vi "Revisión_VFD.vi"(5 "Fabricante":u32, 6 "Modbus":T1, 7 "Iteración (In)":u32, 8 "Motor":T2, 9 "I/O":T3, 10 "Referencias":T4, 11 "Instancia Modbus":refnum<class "Modbus Master.lvclass">) -> (0 "Error Modbus":errorcluster, 2 "Iteración (Out)":u32, 3 "Coincidentes":bool[](array[boolean]))   [LabVIEW 2013]
uses:
  <vilib>/NI/Modbus Library/API/Master/Modbus Master.lvclass
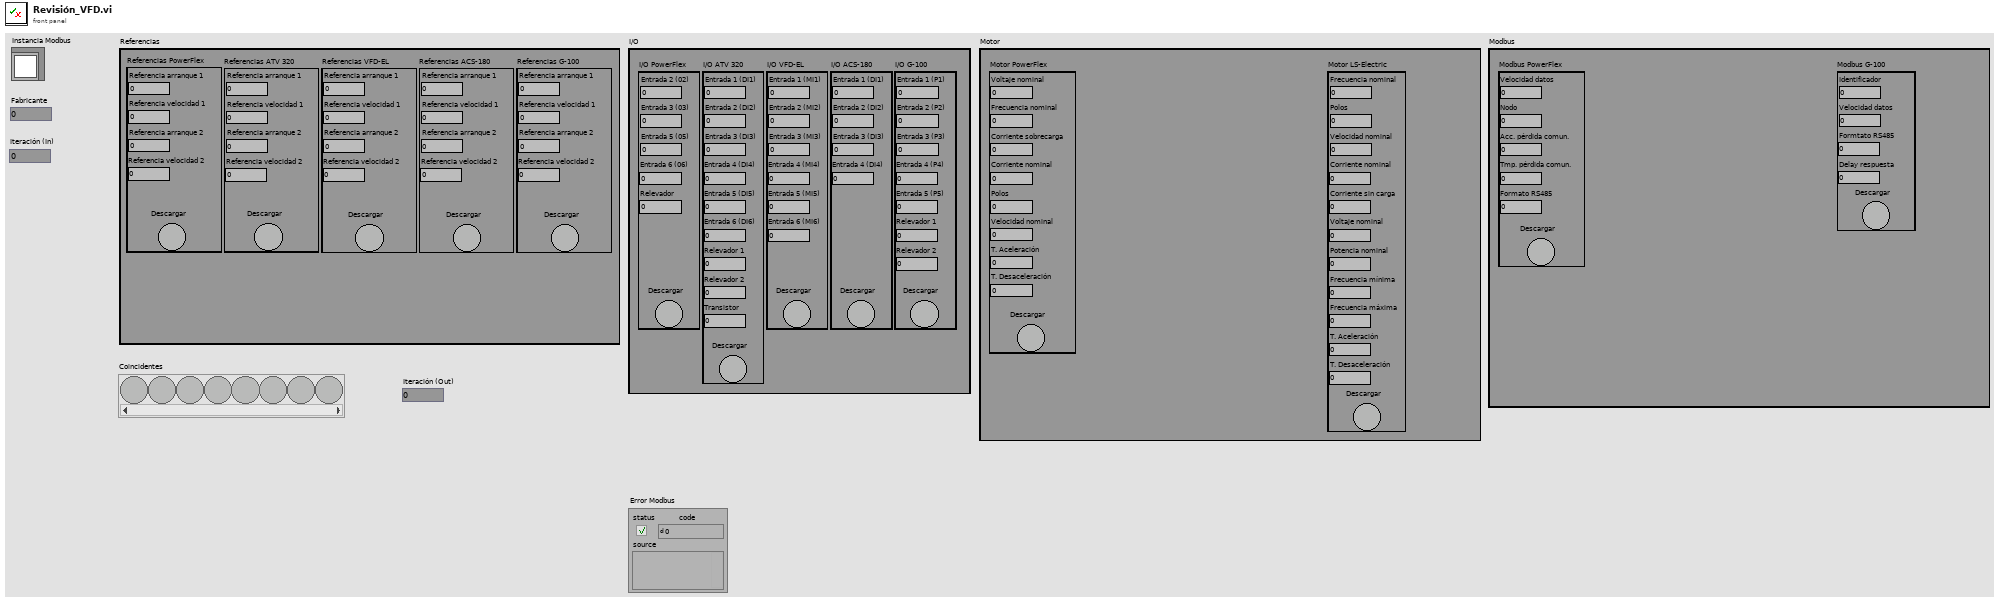
[diagram p1: front panel]
types:
  T1 = cluster{"Modbus PowerFlex":cluster{"Velocidad datos":u16, "Nodo":u16, "Acc. pérdida comun.":u16, "Tmp. pérdida comun.":u16, "Formato RS485":u16, "Descargar":bool}, "Modbus G-100":cluster{"Identificador":u16, "Velocidad datos":u16, "Formtato RS485":u16, "Delay respuesta":u16, "Descargar":bool}}
  T2 = cluster{"Motor PowerFlex":cluster{"Voltaje nominal":u16, "Frecuencia nominal":u16, "Corriente sobrecarga":dbl, "Corriente nominal":dbl, "Polos":u16, "Velocidad nominal":u16, "T. Aceleración":dbl, "T. Desaceleración":dbl, "Descargar":bool}, "Motor LS-Electric":cluster{"Frecuencia nominal":u16, "Polos":u16, "Velocidad nominal":u16, "Corriente nominal":dbl, "Corriente sin carga":dbl, "Voltaje nominal":u16, "Potencia nominal":u16, "Frecuencia mínima":dbl, "Frecuencia máxima":dbl, "T. Aceleración":dbl, "T. Desaceleración":dbl, "Descargar":bool}}
  T3 = cluster{"I/O PowerFlex":cluster{"Entrada 2 (02)":u16, "Entrada 3 (03)":u16, "Entrada 5 (05)":u16, "Entrada 6 (06)":u16, "Relevador":u16, "Descargar":bool}, "I/O ATV 320":cluster{"Entrada 1 (DI1)":u16, "Entrada 2 (DI2)":u16, "Entrada 3 (DI3)":u16, "Entrada 4 (DI4)":u16, "Entrada 5 (DI5)":u16, "Entrada 6 (DI6)":u16, "Relevador 1":u16, "Relevador 2":u16, "Transistor":u16, "Descargar":bool}, "I/O VFD-EL":cluster{"Entrada 1 (MI1)":u16, "Entrada 2 (MI2)":u16, "Entrada 3 (MI3)":u16, "Entrada 4 (MI4)":u16, "Entrada 5 (MI5)":u16, "Entrada 6 (MI6)":u16, "Descargar":bool}, "I/O ACS-180":cluster{"Entrada 1 (DI1)":u16, "Entrada 2 (DI2)":u16, "Entrada 3 (DI3)":u16, "Entrada 4 (DI4)":u16, "Descargar":bool}, "I/O G-100":cluster{"Entrada 1 (P1)":u16, "Entrada 2 (P2)":u16, "Entrada 3 (P3)":u16, "Entrada 4 (P4)":u16, "Entrada 5 (P5)":u16, "Relevador 1":u16, "Relevador 2":u16, "Descargar":bool}}
  T4 = cluster{"Referencias PowerFlex":cluster{"Referencia arranque 1":u16, "Referencia velocidad 1":u16, "Referencia arranque 2":u16, "Referencia velocidad 2":u16, "Descargar":bool}, "Referencias ATV 320":cluster{"Referencia arranque 1":u16, "Referencia velocidad 1":u16, "Referencia arranque 2":u16, "Referencia velocidad 2":u16, "Descargar":bool}, "Referencias VFD-EL":cluster{"Referencia arranque 1":u16, "Referencia velocidad 1":u16, "Referencia arranque 2":u16, "Referencia velocidad 2":u16, "Descargar":bool}, "Referencias ACS-180":cluster{"Referencia arranque 1":u16, "Referencia velocidad 1":u16, "Referencia arranque 2":u16, "Referencia velocidad 2":u16, "Descargar":bool}, "Referencias G-100":cluster{"Referencia arranque 1":u16, "Referencia velocidad 1":u16, "Referencia arranque 2":u16, "Referencia velocidad 2":u16, "Descargar":bool}}
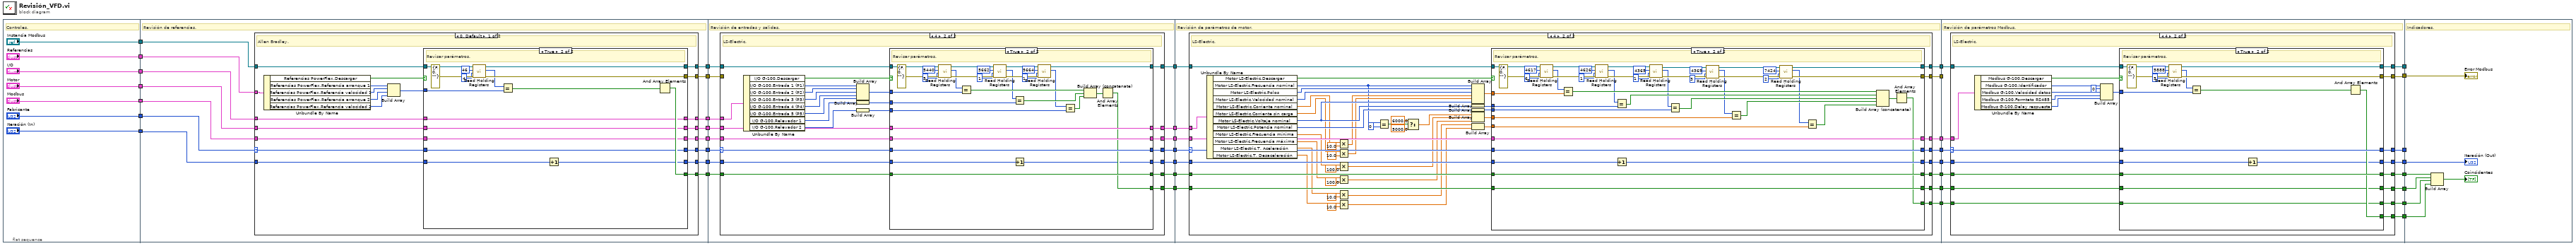
[diagram p0: block diagram]
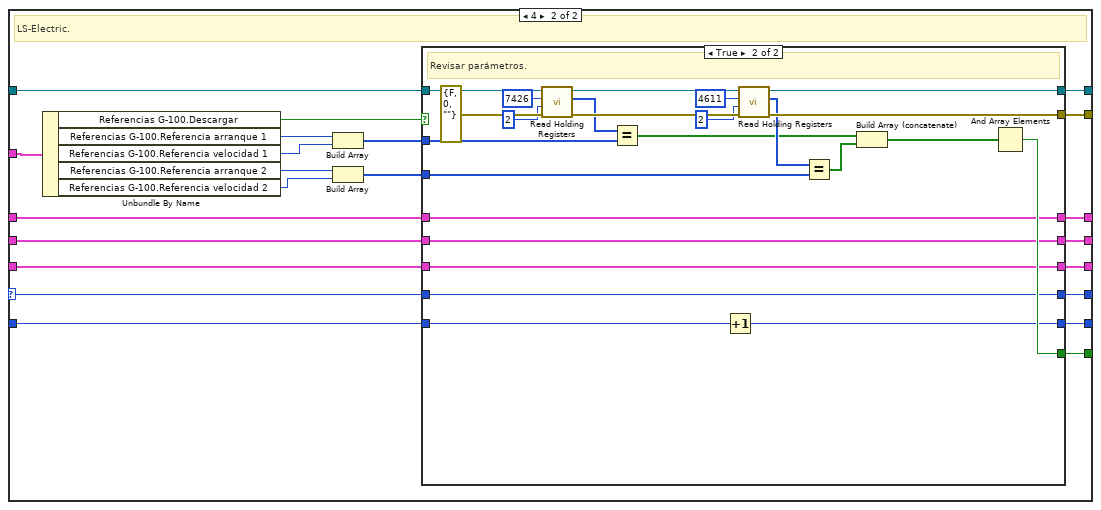
[diagram p3: hidden frame]
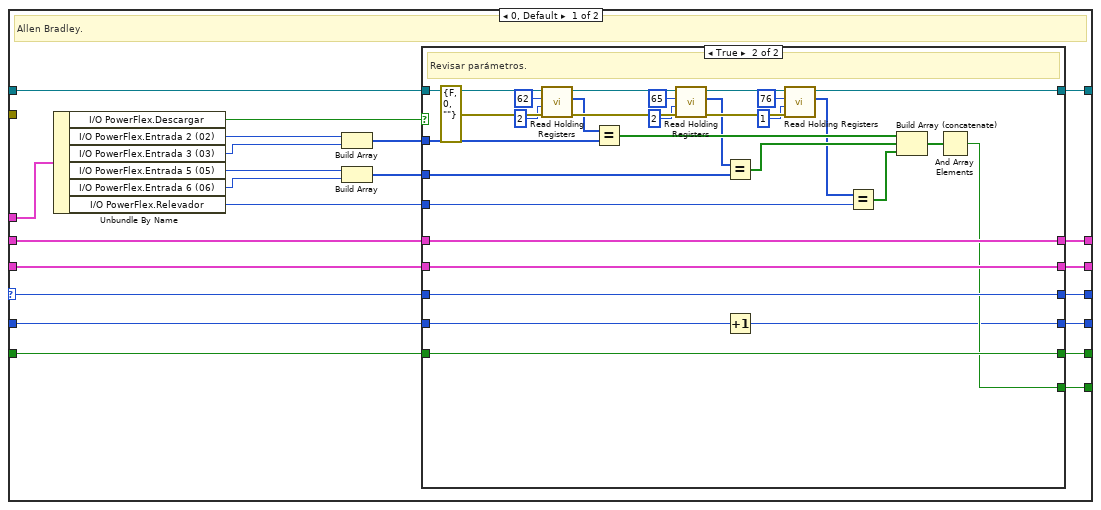
[diagram p5: hidden frame]
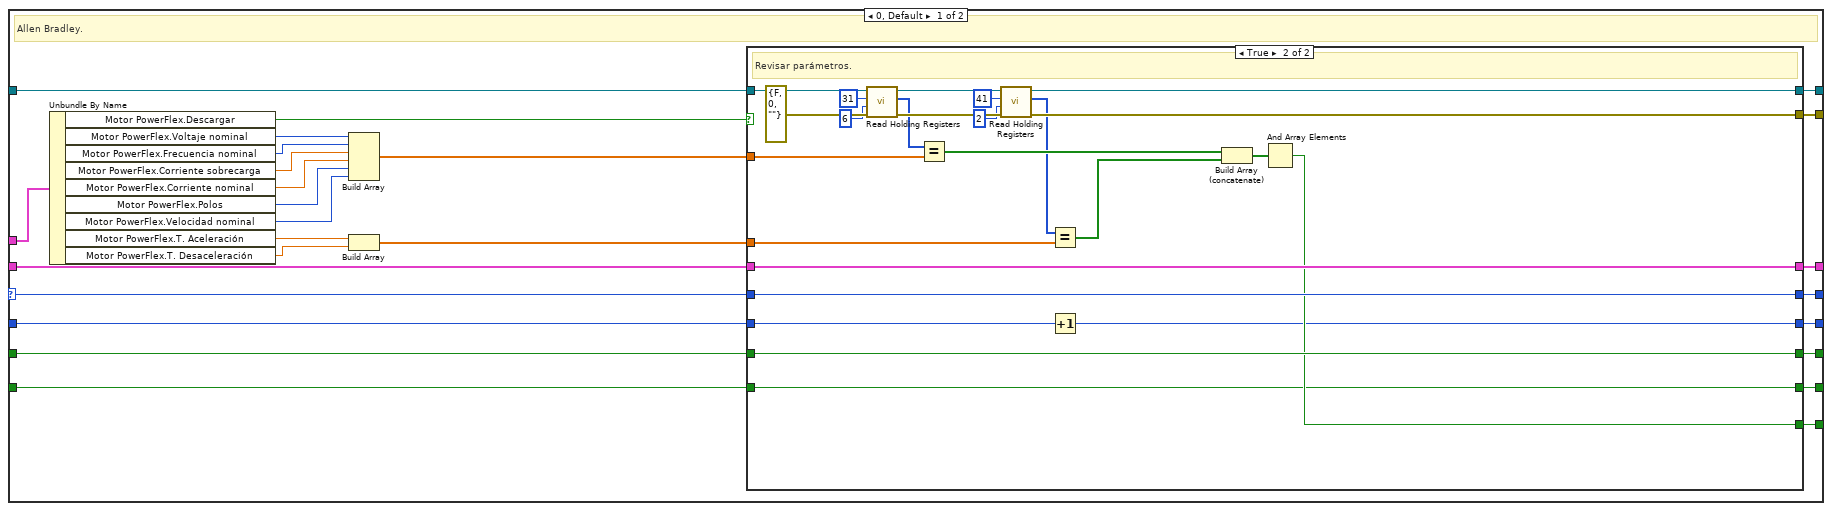
[diagram p8: hidden frame]
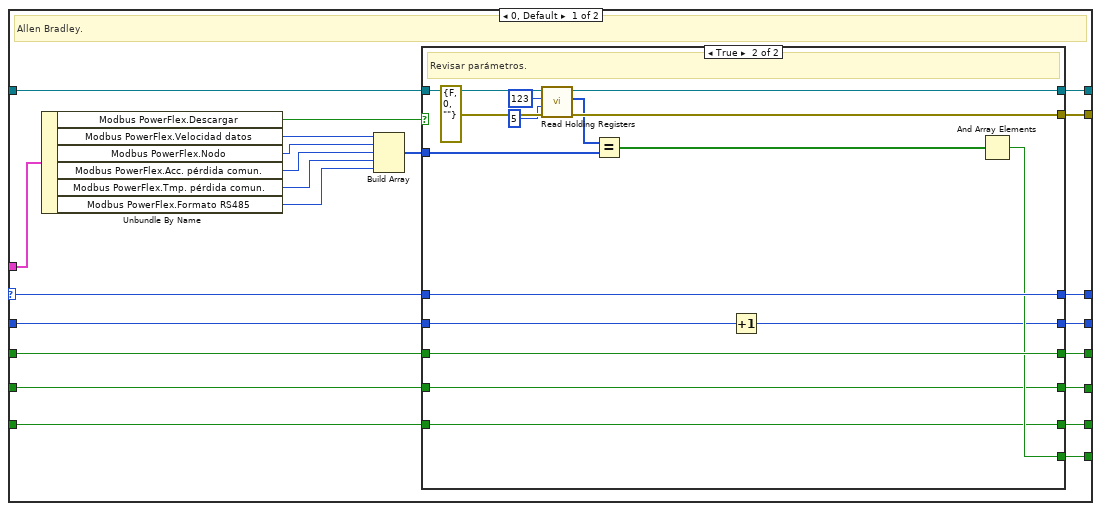
[diagram p11: hidden frame]
diagram:
  n1 = flat-sequence {
    tunnel: ["Instancia Modbus"] -> w38
    tunnel: ["Fabricante"] -> w37
    tunnel: ["Referencias"] -> w36
    tunnel: ["I/O"] -> w35
    tunnel: ["Motor"] -> w34
    tunnel: ["Modbus"] -> w33
    tunnel: ["Iteración (In)"] -> w6
    tunnel: w38 -> [w59]
    tunnel: w37 -> [w60]
    tunnel: w36 -> [w58]
    tunnel: w35 -> [w56]
    tunnel: w34 -> [w55]
    tunnel: w33 -> [w54]
    tunnel: [w57] -> w32
    tunnel: [w53] -> w31
    tunnel: [w52] -> w30
    tunnel: [w51] -> w29
    tunnel: [w50] -> w28
    tunnel: [w49] -> w27
    tunnel: [w48] -> w26
    tunnel: w6 -> [w47]
    tunnel: [w46] -> w5
    tunnel: w32 -> [w164]
    tunnel: w31 -> [w168]
    tunnel: w30 -> [w167]
    tunnel: w29 -> [w166]
    tunnel: w28 -> [w165]
    tunnel: w27 -> [w170]
    tunnel: w26 -> [w169]
    tunnel: [w163] -> w25
    tunnel: [w162] -> w24
    tunnel: [w161] -> w23
    tunnel: [w160] -> w22
    tunnel: [w159] -> w21
    tunnel: [w158] -> w20
    tunnel: w5 -> [w157]
    tunnel: [w156] -> w4
    tunnel: w25 -> [w303]
    tunnel: w24 -> [w302]
    tunnel: w23 -> [w301]
    tunnel: w22 -> [w300]
    tunnel: w21 -> [w299]
    tunnel: w20 -> [w304]
    tunnel: [w298] -> w19
    tunnel: [w297] -> w18
    tunnel: [w296] -> w17
    tunnel: [w295] -> w16
    tunnel: [w294] -> w15
    tunnel: [w293] -> w14
    tunnel: [w292] -> w13
    tunnel: w4 -> [w291]
    tunnel: [w290] -> w3
    tunnel: w19 -> [_]
    tunnel: w18 -> [w475]
    tunnel: w17 -> [w474]
    tunnel: w16 -> [w473]
    tunnel: w15 -> [w472]
    tunnel: w14 -> [w471]
    tunnel: w13 -> [w470]
    tunnel: [w469] -> w12
    tunnel: [w468] -> w11
    tunnel: [w467] -> w10
    tunnel: [w466] -> w9
    tunnel: [w465] -> w8
    tunnel: [w464] -> w7
    tunnel: w3 -> [w463]
    tunnel: [w462] -> w2
    tunnel: [w461] -> w1
    tunnel: w12 -> [_]
    tunnel: w11 -> [w570]
    tunnel: w10 -> [w569]
    tunnel: w9 -> [w568]
    tunnel: w8 -> [w567]
    tunnel: w7 -> [w566]
    tunnel: w2 -> [w564]
    tunnel: w1 -> [_]
    frame #0 {
      # "Controles."
    }
    frame #1 {
      # "Revisión de referencias."
      n2 = case shown="0, Default" w60 {
        selector: w60 -> [w74 w118]
        tunnel: w59 -> [w81 w125]
        tunnel: w58 -> [w80 w124]
        tunnel: [w78 w122] -> w57
        tunnel: w56 -> [w77 w121]
        tunnel: w55 -> [w76 w120]
        tunnel: w54 -> [w75 w119]
        tunnel: [w73 w117] -> w53
        tunnel: [w72 w116] -> w52
        tunnel: [w71 w115] -> w51
        tunnel: [w70 w114] -> w50
        tunnel: [w69 w113] -> w49
        tunnel: [w68 w112] -> w48
        tunnel: w47 -> [w62 w108]
        tunnel: [w61 w107] -> w46
        frame 0, Default {
          # "Allen Bradley."
          n3 = Unbundle By Name(w80) -> ("Referencias PowerFlex.Descargar"=w79:bool, "Referencias PowerFlex.Referencia arranque 1"=w67:u16, "Referencias PowerFlex.Referencia velocidad 1"=w66:u16, "Referencias PowerFlex.Referencia arranque 2"=w65:u16, "Referencias PowerFlex.Referencia velocidad 2"=w64:u16)
          n4 = Build Array(w67, w66, w65, w64) -> (w63:u16[])
          n5 = case shown="True" w79 {
            tunnel: w81 -> [w87 w102]
            tunnel: [_ w96] -> w78
            tunnel: w77 -> [w84 w95]
            tunnel: w76 -> [w83 w94]
            tunnel: w75 -> [w82 w93]
            tunnel: w74 -> [w85 w92]
            tunnel: [w84 w95] -> w73
            tunnel: [w83 w94] -> w72
            tunnel: [w82 w93] -> w71
            tunnel: [w85 w92] -> w70
            tunnel: [w87 w91] -> w69
            tunnel: [_ w103] -> w68
            tunnel: w63 -> [_ w90]
            tunnel: w62 -> [w86 w89]
            tunnel: [w86 w88] -> w61
            frame False {
              # "Nada."
            }
            frame True {
              # "Revisar parámetros."
              n6 = call-dynamic "Read Holding Registers.vi"("error in"=errorcluster {"status"=FALSE, "code"=0, "source"=""}, "number of inputs"=u16 4, "starting address"=u16 46, "Modbus master in"=w102) -> ("error out"=w103:errorcluster, "register values"=w98:u16[], "Modbus master out"=w91:refnum<class "Modbus Master.lvclass">)  [unwired: 5 in]
              n7 = Equal?(x=w98, y=w90) -> (x = y?=w97:bool[])
              n8 = Increment(x=w89) -> (x+1=w88:u32)
              n9 = And Array Elements(Boolean array=w97) -> (logical AND=w96:bool)
            }
          }
        }
        frame 4 {
          # "LS-Electric."
          n10 = Unbundle By Name(w124) -> ("Referencias G-100.Descargar"=w123:bool, "Referencias G-100.Referencia arranque 1"=w111:u16, "Referencias G-100.Referencia velocidad 1"=w110:u16, "Referencias G-100.Referencia arranque 2"=w106:u16, "Referencias G-100.Referencia velocidad 2"=w105:u16)
          n11 = Build Array(w111, w110) -> (w109:u16[])
          n12 = Build Array(w106, w105) -> (w104:u16[])
          n13 = case shown="True" w123 {
            tunnel: w125 -> [w131 w154]
            tunnel: [_ w149] -> w122
            tunnel: w121 -> [w128 w148]
            tunnel: w120 -> [w127 w147]
            tunnel: w119 -> [w126 w146]
            tunnel: w118 -> [w129 w145]
            tunnel: [w128 w148] -> w117
            tunnel: [w127 w147] -> w116
            tunnel: [w126 w146] -> w115
            tunnel: [w129 w145] -> w114
            tunnel: [w131 w139] -> w113
            tunnel: [_ w138] -> w112
            tunnel: w109 -> [_ w144]
            tunnel: w108 -> [w130 w143]
            tunnel: [w130 w142] -> w107
            tunnel: w104 -> [_ w141]
            frame False {
              # "Nada."
            }
            frame True {
              # "Revisar parámetros."
              n14 = call-dynamic "Read Holding Registers.vi"("error in"=errorcluster {"status"=FALSE, "code"=0, "source"=""}, "number of inputs"=u16 2, "starting address"=u16 7426, "Modbus master in"=w154) -> ("error out"=w155:errorcluster, "register values"=w150:u16[], "Modbus master out"=w140:refnum<class "Modbus Master.lvclass">)  [unwired: 5 in]
              n15 = Equal?(x=w150, y=w144) -> (x = y?=w134:bool[])
              n16 = Increment(x=w143) -> (x+1=w142:u32)
              n17 = call-dynamic "Read Holding Registers.vi"("error in"=w155, "number of inputs"=u16 2, "starting address"=u16 4611, "Modbus master in"=w140) -> ("error out"=w138:errorcluster, "register values"=w135:u16[], "Modbus master out"=w139:refnum<class "Modbus Master.lvclass">)  [unwired: 5 in]
              n18 = Equal?(x=w135, y=w141) -> (x = y?=w133:bool[])
              n19 = Build Array (concatenate)(w134, w133) -> (w132:bool[])
              n20 = And Array Elements(Boolean array=w132) -> (logical AND=w149:bool)
            }
          }
        }
      }
    }
    frame #2 {
      # "Revisión de entradas y salidas."
      n21 = case shown="4" w165 {
        selector: w165 -> [w188 w249]
        tunnel: w170 -> [w192 w253]
        tunnel: w168 -> [w184 w245]
        tunnel: w167 -> [w190 w251]
        tunnel: w166 -> [w189 w250]
        tunnel: [w187 w248] -> w163
        tunnel: [w186 w247] -> w162
        tunnel: [w185 w246] -> w161
        tunnel: w169 -> [_ _]
        tunnel: w164 -> [w183 w244]
        tunnel: [w182 w243] -> w160
        tunnel: [w178 w239] -> w158
        tunnel: [w173 w237] -> w159
        tunnel: w157 -> [w172 w236]
        tunnel: [w171 w235] -> w156
        frame 0, Default {
          # "Allen Bradley."
          n22 = Unbundle By Name(w184) -> ("I/O PowerFlex.Descargar"=w191:bool, "I/O PowerFlex.Entrada 2 (02)"=w181:u16, "I/O PowerFlex.Entrada 3 (03)"=w180:u16, "I/O PowerFlex.Entrada 5 (05)"=w177:u16, "I/O PowerFlex.Entrada 6 (06)"=w176:u16, "I/O PowerFlex.Relevador"=w175:u16)
          n23 = Build Array(w181, w180) -> (w179:u16[])
          n24 = Build Array(w177, w176) -> (w174:u16[])
          n25 = case shown="True" w191 {
            tunnel: w192 -> [w198 w225]
            tunnel: w190 -> [w197 w221]
            tunnel: w189 -> [w196 w220]
            tunnel: w188 -> [w195 w219]
            tunnel: [w197 w221] -> w187
            tunnel: [w196 w220] -> w186
            tunnel: [w195 w219] -> w185
            tunnel: [w194 w218] -> w182
            tunnel: w183 -> [w194 w218]
            tunnel: w179 -> [_ w209]
            tunnel: [w198 w213] -> w178
            tunnel: w175 -> [_ w204]
            tunnel: w174 -> [_ w207]
            tunnel: [_ w201] -> w173
            tunnel: w172 -> [w193 w200]
            tunnel: [w193 w199] -> w171
            frame False {
              # "Nada."
            }
            frame True {
              # "Revisar parámetros."
              n26 = call-dynamic "Read Holding Registers.vi"("error in"=errorcluster {"status"=FALSE, "code"=0, "source"=""}, "number of inputs"=u16 2, "starting address"=u16 62, "Modbus master in"=w225) -> ("error out"=w226:errorcluster, "register values"=w210:u16[], "Modbus master out"=w215:refnum<class "Modbus Master.lvclass">)  [unwired: 5 in]
              n27 = Equal?(x=w210, y=w209) -> (x = y?=w227:bool[])
              n28 = call-dynamic "Read Holding Registers.vi"("error in"=w226, "number of inputs"=u16 2, "starting address"=u16 65, "Modbus master in"=w215) -> ("error out"=w212:errorcluster, "register values"=w208:u16[], "Modbus master out"=w214:refnum<class "Modbus Master.lvclass">)  [unwired: 5 in]
              n29 = Equal?(x=w208, y=w207) -> (x = y?=w228:bool[])
              n30 = Increment(x=w200) -> (x+1=w199:u32)
              n31 = call-dynamic "Read Holding Registers.vi"("error in"=w212, "number of inputs"=u16 1, "starting address"=u16 76, "Modbus master in"=w214) -> ("register values"=w205:u16[], "Modbus master out"=w213:refnum<class "Modbus Master.lvclass">)  [unwired: 5 in, 1 out]
              n32 = Equal?(x=w205, y=w204) -> (x = y?=w203:bool[])
              n33 = Build Array (concatenate)(w227, w228, w203) -> (w202:bool[])
              n34 = And Array Elements(Boolean array=w202) -> (logical AND=w201:bool)
            }
          }
        }
        frame 4 {
          # "LS-Electric."
          n35 = Unbundle By Name(w245) -> ("I/O G-100.Descargar"=w252:bool, "I/O G-100.Entrada 1 (P1)"=w242:u16, "I/O G-100.Entrada 2 (P2)"=w241:u16, "I/O G-100.Entrada 3 (P3)"=w234:u16, "I/O G-100.Entrada 4 (P4)"=w233:u16, "I/O G-100.Entrada 5 (P5)"=w232:u16, "I/O G-100.Relevador 1"=w231:u16, "I/O G-100.Relevador 2"=w230:u16)
          n36 = Build Array(w242, w241, w234, w233, w232) -> (w240:u16[])
          n37 = Build Array(w231) -> (w238:u16[])
          n38 = Build Array(w230) -> (w229:u16[])
          n39 = case shown="True" w252 {
            tunnel: w253 -> [w259 w286]
            tunnel: w251 -> [w258 w282]
            tunnel: w250 -> [w257 w281]
            tunnel: w249 -> [w256 w280]
            tunnel: [w258 w282] -> w248
            tunnel: [w257 w281] -> w247
            tunnel: [w256 w280] -> w246
            tunnel: [w255 w279] -> w243
            tunnel: w244 -> [w255 w279]
            tunnel: w240 -> [_ w270]
            tunnel: [w259 w274] -> w239
            tunnel: w238 -> [_ w268]
            tunnel: [_ w263] -> w237
            tunnel: w236 -> [w254 w262]
            tunnel: [w254 w261] -> w235
            tunnel: w229 -> [_ w260]
            frame False {
              # "Nada."
            }
            frame True {
              # "Revisar parámetros."
              n40 = call-dynamic "Read Holding Registers.vi"("error in"=errorcluster {"status"=FALSE, "code"=0, "source"=""}, "number of inputs"=u16 5, "starting address"=u16 5440, "Modbus master in"=w286) -> ("error out"=w287:errorcluster, "register values"=w271:u16[], "Modbus master out"=w276:refnum<class "Modbus Master.lvclass">)  [unwired: 5 in]
              n41 = Equal?(x=w271, y=w270) -> (x = y?=w288:bool[])
              n42 = call-dynamic "Read Holding Registers.vi"("error in"=w287, "number of inputs"=u16 1, "starting address"=u16 5662, "Modbus master in"=w276) -> ("error out"=w273:errorcluster, "register values"=w269:u16[], "Modbus master out"=w275:refnum<class "Modbus Master.lvclass">)  [unwired: 5 in]
              n43 = Equal?(x=w269, y=w268) -> (x = y?=w289:bool[])
              n44 = Increment(x=w262) -> (x+1=w261:u32)
              n45 = call-dynamic "Read Holding Registers.vi"("error in"=w273, "number of inputs"=u16 1, "starting address"=u16 5664, "Modbus master in"=w275) -> ("register values"=w266:u16[], "Modbus master out"=w274:refnum<class "Modbus Master.lvclass">)  [unwired: 5 in, 1 out]
              n46 = Equal?(x=w266, y=w260) -> (x = y?=w265:bool[])
              n47 = Build Array (concatenate)(w288, w289, w265) -> (w264:bool[])
              n48 = And Array Elements(Boolean array=w264) -> (logical AND=w263:bool)
            }
          }
        }
      }
    }
    frame #3 {
      # "Revisión de parámetros de motor."
      n49 = case shown="4" w301 {
        selector: w301 -> [w327 w405]
        tunnel: w304 -> [w330 w408]
        tunnel: w303 -> [w320 w398]
        tunnel: w302 -> [w328 w406]
        tunnel: [w326 w404] -> w296
        tunnel: [w325 w403] -> w295
        tunnel: w300 -> [w324 w402]
        tunnel: [w323 w401] -> w294
        tunnel: [w322 w400] -> w297
        tunnel: [w321 w399] -> w293
        tunnel: w299 -> [w308 w391]
        tunnel: [w309 w392] -> w298
        tunnel: [w307 w390] -> w292
        tunnel: w291 -> [w306 w389]
        tunnel: [w305 w388] -> w290
        frame 0, Default {
          # "Allen Bradley."
          n50 = Unbundle By Name(w320) -> ("Motor PowerFlex.Descargar"=w329:bool, "Motor PowerFlex.Voltaje nominal"=w319:u16, "Motor PowerFlex.Frecuencia nominal"=w318:u16, "Motor PowerFlex.Corriente sobrecarga"=w317:dbl, "Motor PowerFlex.Corriente nominal"=w316:dbl, "Motor PowerFlex.Polos"=w315:u16, "Motor PowerFlex.Velocidad nominal"=w314:u16, "Motor PowerFlex.T. Aceleración"=w312:dbl, "Motor PowerFlex.T. Desaceleración"=w311:dbl)
          n51 = Build Array(w319, w318, w317, w316, w315, w314) -> (w313:dbl[])
          n52 = Build Array(w312, w311) -> (w310:dbl[])
          n53 = case shown="True" w329 {
            tunnel: w330 -> [w336 w356]
            tunnel: w328 -> [w335 w352]
            tunnel: w327 -> [w334 w351]
            tunnel: [w335 w352] -> w326
            tunnel: [w334 w351] -> w325
            tunnel: [w333 w350] -> w323
            tunnel: w324 -> [w333 w350]
            tunnel: [w336 w340] -> w322
            tunnel: [_ w343] -> w321
            tunnel: w313 -> [_ w342]
            tunnel: w310 -> [_ w341]
            tunnel: [_ w360] -> w309
            tunnel: w308 -> [w332 w339]
            tunnel: [w332 w339] -> w307
            tunnel: w306 -> [w331 w338]
            tunnel: [w331 w337] -> w305
            frame False {
              # "Nada."
            }
            frame True {
              # "Revisar parámetros."
              n54 = call-dynamic "Read Holding Registers.vi"("error in"=errorcluster {"status"=FALSE, "code"=0, "source"=""}, "number of inputs"=u16 6, "starting address"=u16 31, "Modbus master in"=w356) -> ("error out"=w357:errorcluster, "register values"=w346:u16[], "Modbus master out"=w347:refnum<class "Modbus Master.lvclass">)  [unwired: 5 in]
              n55 = Equal?(x=w346, y=w342) -> (x = y?=w358:bool[])
              n56 = call-dynamic "Read Holding Registers.vi"("error in"=w357, "number of inputs"=u16 2, "starting address"=u16 41, "Modbus master in"=w347) -> ("error out"=w360:errorcluster, "register values"=w345:u16[], "Modbus master out"=w340:refnum<class "Modbus Master.lvclass">)  [unwired: 5 in]
              n57 = Equal?(x=w345, y=w341) -> (x = y?=w359:bool[])
              n58 = Increment(x=w338) -> (x+1=w337:u32)
              n59 = Build Array (concatenate)(w358, w359) -> (w344:bool[])
              n60 = And Array Elements(Boolean array=w344) -> (logical AND=w343:bool)
            }
          }
        }
        frame 4 {
          # "LS-Electric."
          n61 = Unbundle By Name(w398) -> ("Motor LS-Electric.Descargar"=w407:bool, "Motor LS-Electric.Frecuencia nominal"=w366:u16, "Motor LS-Electric.Polos"=w397:u16, "Motor LS-Electric.Velocidad nominal"=w396:u16, "Motor LS-Electric.Corriente nominal"=w386:dbl, "Motor LS-Electric.Corriente sin carga"=w383:dbl, "Motor LS-Electric.Voltaje nominal"=w409:u16, "Motor LS-Electric.Potencia nominal"=w394:u16, "Motor LS-Electric.Frecuencia mínima"=w376:dbl, "Motor LS-Electric.Frecuencia máxima"=w373:dbl, "Motor LS-Electric.T. Aceleración"=w370:dbl, "Motor LS-Electric.T. Desaceleración"=w362:dbl)
          n62 = Multiply(x=w386, y=10.0) -> (x*y=w385:dbl)
          n63 = Multiply(x=w383, y=10.0) -> (x*y=w382:dbl)
          n64 = Multiply(x=w376, y=100.0) -> (x*y=w375:dbl)
          n65 = Multiply(x=w373, y=100.0) -> (x*y=w372:dbl)
          n66 = Multiply(x=w370, y=10.0) -> (x*y=w365:dbl)
          n67 = Multiply(x=w362, y=10.0) -> (x*y=w361:dbl)
          n68 = Equal?(x=w366, y=u16 0) -> (x = y?=w367:bool)
          n69 = Select(t=6000.0, s=w367, f=5000.0) -> (s? t:f=w378:dbl)
          n70 = Build Array(w366, w397, w396, w385, w382, w409) -> (w395:dbl[])
          n71 = Build Array(w409) -> (w381:u16[])
          n72 = Build Array(w394) -> (w393:u16[])
          n73 = Build Array(w378, w375, w372) -> (w369:dbl[])
          n74 = Build Array(w365, w361) -> (w364:dbl[])
          n75 = case shown="True" w407 {
            tunnel: w408 -> [w415 w454]
            tunnel: w406 -> [w414 w450]
            tunnel: w405 -> [w413 w449]
            tunnel: [w414 w450] -> w404
            tunnel: [w413 w449] -> w403
            tunnel: [w412 w448] -> w401
            tunnel: w402 -> [w412 w448]
            tunnel: [w415 w424] -> w400
            tunnel: [_ w419] -> w399
            tunnel: w395 -> [_ w441]
            tunnel: w393 -> [_ w432]
            tunnel: [_ w423] -> w392
            tunnel: w391 -> [w411 w440]
            tunnel: [w411 w440] -> w390
            tunnel: w389 -> [w410 w439]
            tunnel: [w410 w438] -> w388
            tunnel: w381 -> [_ w437]
            tunnel: w369 -> [_ w421]
            tunnel: w364 -> [_ w416]
            frame False {
              # "Nada."
            }
            frame True {
              # "Revisar parámetros."
              n76 = call-dynamic "Read Holding Registers.vi"("error in"=errorcluster {"status"=FALSE, "code"=0, "source"=""}, "number of inputs"=u16 6, "starting address"=u16 4617, "Modbus master in"=w454) -> ("error out"=w455:errorcluster, "register values"=w444:u16[], "Modbus master out"=w445:refnum<class "Modbus Master.lvclass">)  [unwired: 5 in]
              n77 = Equal?(x=w444, y=w441) -> (x = y?=w456:bool[])
              n78 = call-dynamic "Read Holding Registers.vi"("error in"=w455, "number of inputs"=u16 1, "starting address"=u16 4626, "Modbus master in"=w445) -> ("error out"=w458:errorcluster, "register values"=w443:u16[], "Modbus master out"=w434:refnum<class "Modbus Master.lvclass">)  [unwired: 5 in]
              n79 = Equal?(x=w443, y=w437) -> (x = y?=w457:bool[])
              n80 = Increment(x=w439) -> (x+1=w438:u32)
              n81 = call-dynamic "Read Holding Registers.vi"("error in"=w458, "number of inputs"=u16 1, "starting address"=u16 4365, "Modbus master in"=w434) -> ("error out"=w459:errorcluster, "register values"=w433:u16[], "Modbus master out"=w426:refnum<class "Modbus Master.lvclass">)  [unwired: 5 in]
              n82 = Equal?(x=w433, y=w432) -> (x = y?=w431:bool[])
              n83 = call-dynamic "Read Holding Registers.vi"("error in"=w459, "number of inputs"=u16 3, "starting address"=u16 4369, "Modbus master in"=w426) -> ("error out"=w460:errorcluster, "register values"=w422:u16[], "Modbus master out"=w425:refnum<class "Modbus Master.lvclass">)  [unwired: 5 in]
              n84 = Equal?(x=w422, y=w421) -> (x = y?=w420:bool[])
              n85 = call-dynamic "Read Holding Registers.vi"("error in"=w460, "number of inputs"=u16 2, "starting address"=u16 7424, "Modbus master in"=w425) -> ("error out"=w423:errorcluster, "register values"=w418:u16[], "Modbus master out"=w424:refnum<class "Modbus Master.lvclass">)  [unwired: 5 in]
              n86 = Equal?(x=w418, y=w416) -> (x = y?=w417:bool[])
              n87 = Build Array (concatenate)(w456, w457, w431, w420, w417) -> (w442:bool[])
              n88 = And Array Elements(Boolean array=w442) -> (logical AND=w419:bool)
            }
          }
        }
      }
    }
    frame #4 {
      # "Revisión de parámetros Modbus."
      n89 = case shown="4" w473 {
        selector: w473 -> [w495 w539]
        tunnel: w475 -> [w497 w541]
        tunnel: w474 -> [w487 w531]
        tunnel: [w494 w538] -> w461
        tunnel: w472 -> [w493 w537]
        tunnel: [w492 w536] -> w467
        tunnel: [w491 w535] -> w469
        tunnel: [w490 w534] -> w464
        tunnel: [w488 w532] -> w468
        tunnel: w471 -> [w485 w529]
        tunnel: w470 -> [w486 w530]
        tunnel: [w479 w527] -> w466
        tunnel: [w478 w526] -> w465
        tunnel: w463 -> [w477 w525]
        tunnel: [w476 w524] -> w462
        frame 0, Default {
          # "Allen Bradley."
          n90 = Unbundle By Name(w487) -> ("Modbus PowerFlex.Descargar"=w496:bool, "Modbus PowerFlex.Velocidad datos"=w484:u16, "Modbus PowerFlex.Nodo"=w483:u16, "Modbus PowerFlex.Acc. pérdida comun."=w482:u16, "Modbus PowerFlex.Tmp. pérdida comun."=w481:u16, "Modbus PowerFlex.Formato RS485"=w480:u16)
          n91 = Build Array(w484, w483, w482, w481, w480) -> (w489:u16[])
          n92 = case shown="True" w496 {
            tunnel: w497 -> [w503 w518]
            tunnel: w495 -> [w502 w514]
            tunnel: [w502 w514] -> w494
            tunnel: [w501 w513] -> w492
            tunnel: w493 -> [w501 w513]
            tunnel: [w503 w509] -> w491
            tunnel: [_ w511] -> w490
            tunnel: w489 -> [_ w510]
            tunnel: [_ w519] -> w488
            tunnel: w486 -> [w500 w507]
            tunnel: w485 -> [w499 w506]
            tunnel: [w500 w507] -> w479
            tunnel: [w499 w506] -> w478
            tunnel: w477 -> [w498 w505]
            tunnel: [w498 w504] -> w476
            frame False {
              # "Nada."
            }
            frame True {
              # "Revisar parámetros."
              n93 = call-dynamic "Read Holding Registers.vi"("error in"=errorcluster {"status"=FALSE, "code"=0, "source"=""}, "number of inputs"=u16 5, "starting address"=u16 123, "Modbus master in"=w518) -> ("error out"=w519:errorcluster, "register values"=w512:u16[], "Modbus master out"=w509:refnum<class "Modbus Master.lvclass">)  [unwired: 5 in]
              n94 = Equal?(x=w512, y=w510) -> (x = y?=w508:bool[])
              n95 = Increment(x=w505) -> (x+1=w504:u32)
              n96 = And Array Elements(Boolean array=w508) -> (logical AND=w511:bool)
            }
          }
        }
        frame 4 {
          # "LS-Electric."
          n97 = Unbundle By Name(w531) -> ("Modbus G-100.Descargar"=w540:bool, "Modbus G-100.Identificador"=w528:u16, "Modbus G-100.Velocidad datos"=w523:u16, "Modbus G-100.Formtato RS485"=w522:u16, "Modbus G-100.Delay respuesta"=w521:u16)
          n98 = Build Array(w528, u16 0 ("element"), w523, w522, w521) -> (w533:u16[])
          n99 = case shown="True" w540 {
            tunnel: w541 -> [w547 w562]
            tunnel: w539 -> [w546 w558]
            tunnel: [w546 w558] -> w538
            tunnel: [w545 w557] -> w536
            tunnel: w537 -> [w545 w557]
            tunnel: [w547 w553] -> w535
            tunnel: [_ w555] -> w534
            tunnel: w533 -> [_ w554]
            tunnel: [_ w563] -> w532
            tunnel: w530 -> [w544 w551]
            tunnel: w529 -> [w543 w550]
            tunnel: [w544 w551] -> w527
            tunnel: [w543 w550] -> w526
            tunnel: w525 -> [w542 w549]
            tunnel: [w542 w548] -> w524
            frame False {
              # "Nada."
            }
            frame True {
              # "Revisar parámetros."
              n100 = call-dynamic "Read Holding Registers.vi"("error in"=errorcluster {"status"=FALSE, "code"=0, "source"=""}, "number of inputs"=u16 5, "starting address"=u16 5888, "Modbus master in"=w562) -> ("error out"=w563:errorcluster, "register values"=w556:u16[], "Modbus master out"=w553:refnum<class "Modbus Master.lvclass">)  [unwired: 5 in]
              n101 = Equal?(x=w556, y=w554) -> (x = y?=w552:bool[])
              n102 = Increment(x=w549) -> (x+1=w548:u32)
              n103 = And Array Elements(Boolean array=w552) -> (logical AND=w555:bool)
            }
          }
        }
      }
    }
    frame #5 {
      # "Indicadores."
      n104 = Build Array(w569, w568, w567, w566) -> (→"Coincidentes":bool[])
      "Error Modbus" <- w570
      "Iteración (Out)" <- w564
    }
  }
